vi "Parse Response.vi"(8 "error in (no error)":errorcluster, 9 "Command":string, 10 "Response":string, 11 "VISA resource in":refnum<visa-resource-name>) -> (0 "error out":errorcluster, 2 "Information":string, 3 "VISA resource out":refnum<visa-resource-name>)   [LabVIEW 2020, in "Global FIA milliGAT.lvlib"]
doc: "Checks if the response contains the original command, that the message was valid, and returns any information prompted for by the message."
uses:
  <instrlib>/RxnRover/Global FIA milliGAT 3.14/Global FIA milliGAT.lvlib
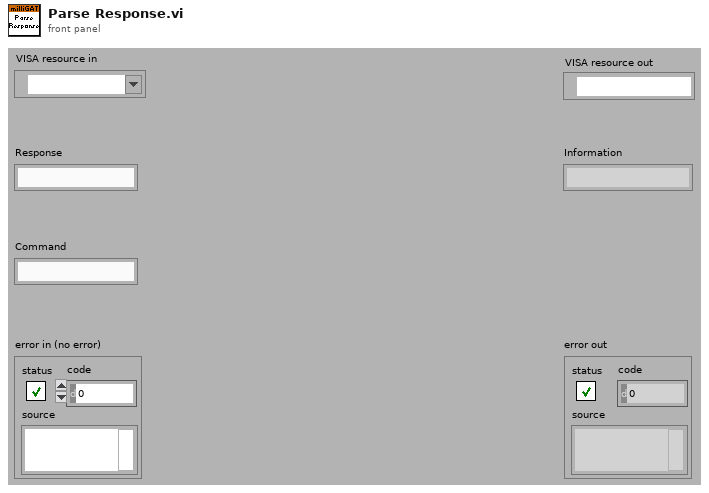
[diagram p1: front panel]
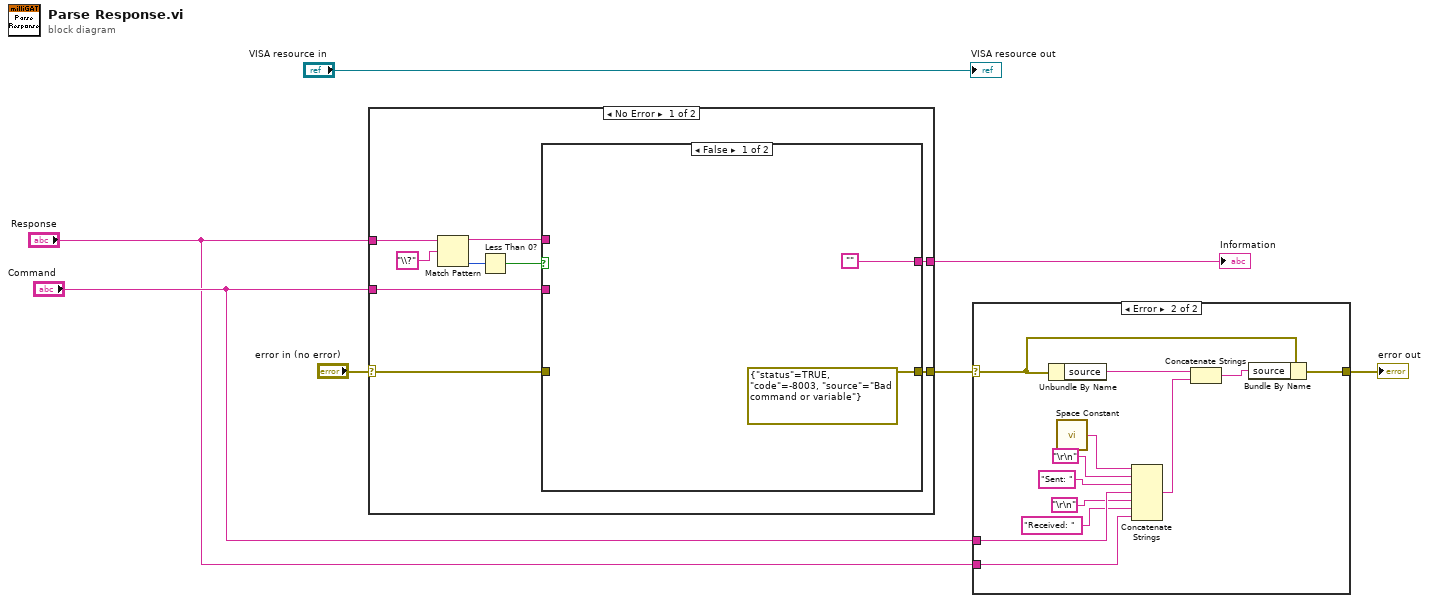
[diagram p0: block diagram]
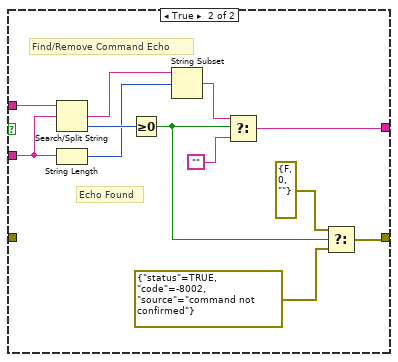
[diagram p3: hidden frame]
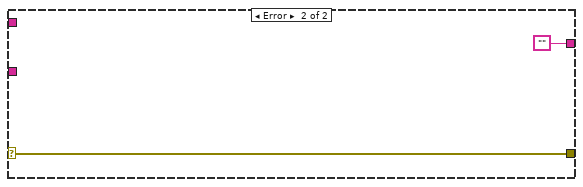
[diagram p4: hidden frame]
diagram:
  n1 = case shown="No Error" "error in (no error)" {
    selector: "error in (no error)" -> [w11 w32]
    tunnel: "Response" -> [w16 _]
    tunnel: [w10 w32] -> w4
    tunnel: [w9 ""] -> w6
    tunnel: "Command" -> [w8 _]
    frame No Error {
      n2 = Match Pattern(string=w16, regular expression="\\?") -> (before substring=w12:string, offset past match=w13:i32)  [unwired: 1 in, 2 out]
      n3 = Less Than 0?(x=w13) -> (x < 0?=w14:bool)
      n4 = case shown="False" w14 {
        tunnel: w12 -> [_ w22]
        tunnel: w11 -> [_ _]
        tunnel: [errorcluster {"status"=TRUE, "code"=-8003, "source"="Bad command or variable"} ("error IO") w30] -> w10
        tunnel: ["" w20] -> w9
        tunnel: w8 -> [_ w21]
        frame False {
        }
        frame True {
          # "Echo Found"
          # "Find/Remove Command Echo"
          n5 = Search/Split String(string=w22, search string/char (-)=w21) -> (match + rest of string=w26:string, offset of match=w27:i32)  [unwired: 1 in, 1 out]
          n6 = String Length(string=w21) -> (length=w25:i32)
          n7 = Greater Or Equal To 0?(x=w27) -> (x >= 0?=w19:bool)
          n8 = String Subset(string=w26, offset (0)=w25) -> (substring=w24:string)  [unwired: 1 in]
          n9 = Select(t=w24, s=w19, f="") -> (s? t:f=w20:string)
          n10 = Select(t=errorcluster {"status"=FALSE, "code"=0, "source"=""} ("f"), s=w19, f=errorcluster {"status"=TRUE, "code"=-8002, "source"="command not confirmed"} ("error IO")) -> (s? t:f=w30:errorcluster)
        }
      }
    }
    frame Error {
    }
  }
  "Information" <- w6
  n11 = case shown="Error" w4 {
    selector: w4 -> [w33 w36]
    tunnel: "Command" -> [_ w42]
    tunnel: "Response" -> [_ w39]
    tunnel: [w33 w34] -> w1
    frame No Error {
    }
    frame Error {
      n12 = Unbundle By Name(w36) -> ("source"=w38:string)
      n13 = call <vilib>:"Space Constant.vi"() -> ("String"=w45:string)
      n14 = Concatenate Strings(w45, "\r\n", "Sent: " ("string"), w42, "\r\n", "Received: " ("string"), w39) -> (w37:string)
      n15 = Concatenate Strings(w38, w37) -> (w35:string)
      n16 = Bundle By Name(cluster=w36, "source"=w35) -> (w34:errorcluster)
    }
  }
  "error out" <- w1
  "VISA resource out" <- "VISA resource in"
